vi "History Read.vi"(4 "error in (no error)":errorcluster, 6 "Container State":T2, 7 "Display State In":T1 {"Time" format="%<%H:%M:%S>T"}) -> (0 "error out":errorcluster, 2 "Value":i32, 3 "Display State Out":T1 {"Time" format="%<%H:%M:%S>T"})   [LabVIEW 2015, in "1D Xctl Buffer.xctl"]
uses:
  1D Xctl Buffer.xctl
  <vilib>/_xctls/Container State.ctl
  1D Buffer State.ctl
  <vilib>/_xctls/XControlSupport.lvlib
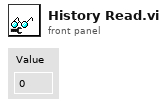
[diagram p1: front panel]
types:
  T1 = typedef "1D Xctl Buffer.xctl/1D Buffer State.ctl" = cluster{"History":i32, "Time":timestamp[], "Data":u16[]}
  T2 = typedef "XControlSupport.lvlib/Container State.ctl" = cluster{"Indicator?":bool, "Run Mode?":bool, " Refnum":refnum<vi>}
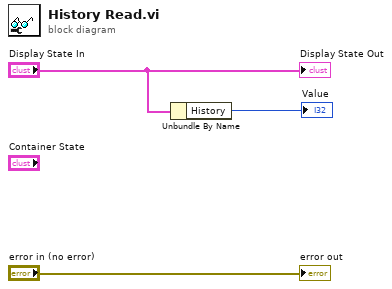
[diagram p0: block diagram]
diagram:
  n1 = Unbundle By Name("Display State In") -> ("History"=→"Value":i32)
  "error out" <- "error in (no error)"
  "Display State Out" <- "Display State In"
